vi "Set default values.vi"(8 "error in (no error)":errorcluster, 11 "device data model in":refnum<class "ICPCON PM3114 Data Model.lvclass">) -> (0 "error out":errorcluster, 3 "device data model out":refnum<class "ICPCON PM3114 Data Model.lvclass">)   [LabVIEW 2021, in "ICPCON PM3114 Data Model.lvclass"]
doc: "This VI ensures that the data model has at least 65,535 values of every type. This is required for certain modbus function codes."
uses:
  ICPCON PM3114 Data Model.lvclass
  ICPCON PM3114 Data Model.lvclass/ICPCON PM3114 Data Model.ctl
  Type Definitions/Data Model.ctl
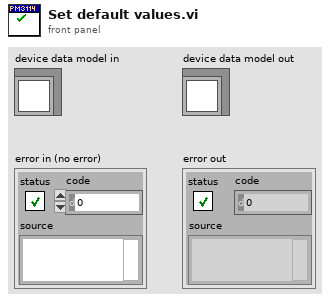
[diagram p1: front panel]
types:
  T1 = typedef "ICPCON PM3114 Data Model.lvclass/Data Model.ctl" = cluster{"UTC":u64, "Power value":sgl[], "ES":u8}
  T2 = typedef "Device Data Model.lvclass/N channel.ctl" = cluster{"N DI channel":i32, "N DO channel":i32, "N AI channel":i32, "N AO channel":i32}
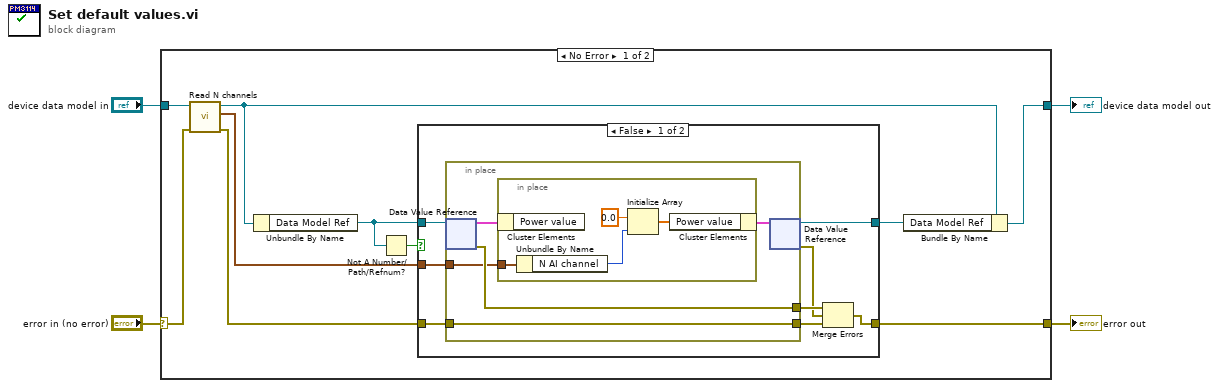
[diagram p0: block diagram]
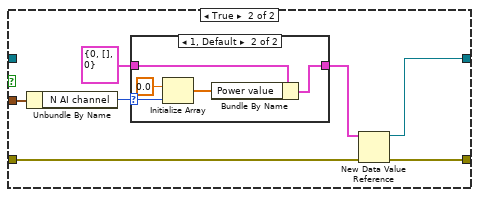
[diagram p2: hidden frame]
diagram:
  n1 = case shown="No Error" "error in (no error)" {
    selector: "error in (no error)" -> [w7 w46]
    tunnel: "device data model in" -> [w9 w45]
    tunnel: [w14 w45] -> w3
    tunnel: [w10 w46] -> w2
    frame No Error {
      n2 = call-dynamic "Read N channels.vi"("error in (no error)"=w7, "device data model in"=w9) -> ("error out"=w6:errorcluster, "N channel"=w5:T2, "device data model out"=w8:refnum<class "ICPCON PM3114 Data Model.lvclass">)  [unwired: 7 in]
      n3 = Unbundle By Name(w8) -> ("Data Model Ref"=w12:refnum<data-value>)
      n4 = Not A Number/Path/Refnum?(number/path/refnum=w12) -> (NaN/Path/Refnum?=w11:bool)
      n5 = case shown="False" w11 {
        tunnel: w6 -> [w22 w38]
        tunnel: w12 -> [w21 _]
        tunnel: [w20 w36] -> w13
        tunnel: [w18 w37] -> w10
        tunnel: w5 -> [w15 w33]
        frame False {
          n6 = in-place {
            in-place-border: w22 -> [w25]
            in-place-border: [w26] -> w19
            in-place-border: [w25] -> w16
            in-place-border: w15 -> [w24]
            n7 = in-place-dvr #1(w21) -> (w27:T1, w26:errorcluster)
            n8 = in-place {
              in-place-border: w24 -> [w30]
              n9 = in-place-cluster #2(w27) -> ()  [unwired: 1 out]
              n10 = Unbundle By Name(w30) -> ("N AI channel"=w29:i32)
              n11 = Initialize Array(sgl 0.0 ("Boolean"), w29) -> (w28:sgl[])
              n12 = in-place-cluster #2("Power value"=w28) -> (w23:T1)
            }
            n13 = in-place-dvr #1(w23) -> (w20:refnum<data-value>, w17:errorcluster)
          }
          n14 = Merge Errors(w19, w17, w16) -> (w18:errorcluster)
        }
        frame True {
          n15 = Unbundle By Name(w33) -> ("N AI channel"=w34:i32)
          n16 = case shown="1, Default" w34 {
            selector: w34 -> [_ w40]
            tunnel: T1 {"UTC"=0, "Power value"=[], "ES"=0} ("Data Model") -> [w39 w43]
            tunnel: [w39 w41] -> w32
            frame 0 {
            }
            frame 1, Default {
              n17 = Initialize Array(sgl 0.0 ("Boolean"), w40) -> (w42:sgl[])
              n18 = Bundle By Name(cluster=w43, "Power value"=w42) -> (w41:T1)
            }
          }
          n19 = New Data Value Reference(data value=w32, error in=w38) -> (data value reference=w36:refnum<data-value>, error out=w37:errorcluster)
        }
      }
      n20 = Bundle By Name(cluster=w8, "Data Model Ref"=w13) -> (w14:refnum<class "ICPCON PM3114 Data Model.lvclass">)
    }
    frame Error {
    }
  }
  "error out" <- w2
  "device data model out" <- w3
